vi "ValidateRule.vi"(8 "error in (no error)":errorcluster, 9 "Target":refnum<class "ILabVIEWItem.lvclass">, 11 "CDependencyItemRule in":refnum<class "CDependencyItemRule.lvclass">) -> (0 "error out":errorcluster, 1 "Pass?":bool, 2 "Is concession?":bool, 3 "CDependencyItemRule out":refnum<class "CDependencyItemRule.lvclass">)   [LabVIEW 2020, in "LabVIEWContainers.lvlib" / "CDependencyItemRule.lvclass"]
uses:
  CDependencyItemRule.lvclass
  LabVIEWObjectInterfaces/ILabVIEWItem/ILabVIEWItem.lvclass
  CommonHelpers/CommonHelpers.lvlib
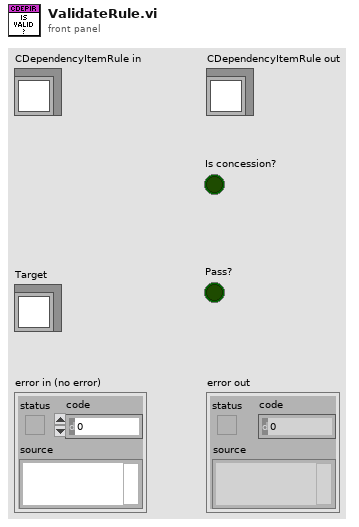
[diagram p1: front panel]
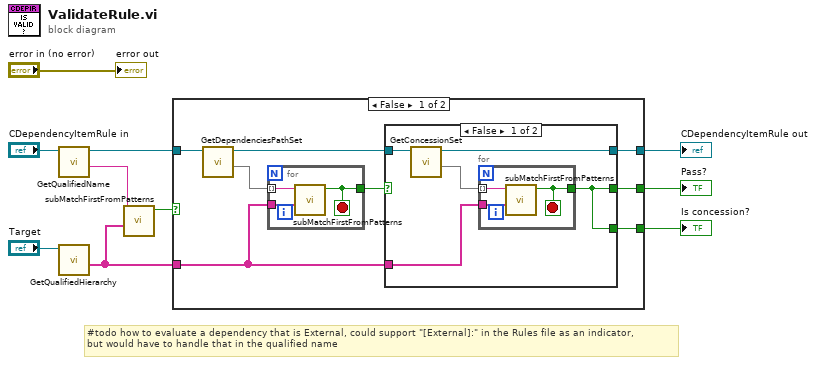
[diagram p0: block diagram]
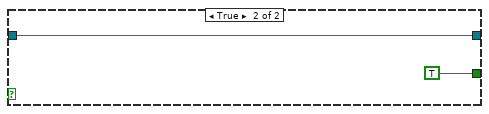
[diagram p3: hidden frame]
diagram:
  # "#todo how to evaluate a dependency that is External, could support \"[External]:\" in the Rules file as an indicator, \nbut would have to handle that in the qualified name"
  n1 = call-dynamic "GetQualifiedName.vi"("CLabVIEWItem in"="CDependencyItemRule in") -> ("Qualified name"=w3:string, "CLabVIEWItem out"=w4:refnum<class "CDependencyItemRule.lvclass">)  [unwired: 8 in, 1 out]
  n2 = call-dynamic "GetQualifiedHierarchy.vi"("ILabVIEWItem in"="Target") -> ("Qualified hierarchy"=w2:string[])  [unwired: 8 in, 2 out]
  n3 = call "subMatchFirstFromPatterns.vi"("patterns"=w2, "string in"=w3) -> ("found?"=w1:bool)  [unwired: 7 in, 2 out]
  n4 = case shown="False" w1 {
    tunnel: w4 -> [w18 w33]
    tunnel: [w16 w33] -> w9
    tunnel: [w13 TRUE ("found?")] -> w7
    tunnel: [w12 _] -> w6
    tunnel: w2 -> [w11 _]
    frame False {
      n5 = call-dynamic "GetDependenciesPathSet.vi"("CLabVIEWItem in"=w18) -> ("Dependencies"=w15:set{string}, "CLabVIEWItem out"=w17:refnum<class "CDependencyItemRule.lvclass">)  [unwired: 8 in, 1 out]
      n6 = for {
        tunnel: w15 -> [w31] mode=indexing
        tunnel: w11 -> [w30]
        tunnel: [w29] -> w14
        stop <- w29 stop-if-true
        n7 = call "subMatchFirstFromPatterns.vi"("patterns"=w30, "string in"=w31) -> ("found?"=w29:bool)  [unwired: 7 in, 2 out]
      }
      n8 = case shown="False" w14 {
        selector: w14 -> [_ w27]
        tunnel: w17 -> [w23 w28]
        tunnel: [w22 w28] -> w16
        tunnel: w11 -> [w20 _]
        tunnel: [w19 w27] -> w13
        tunnel: [w19 _] -> w12
        frame False {
          n9 = call-dynamic "GetConcessionSet.vi"("CDependencyItemRule in"=w23) -> ("Concessions"=w21:set{string}, "CDependencyItemRule out"=w22:refnum<class "CDependencyItemRule.lvclass">)  [unwired: 8 in, 1 out]
          n10 = for {
            tunnel: w21 -> [w26] mode=indexing
            tunnel: w20 -> [w25]
            tunnel: [w24] -> w19
            stop <- w24 stop-if-true
            n11 = call "subMatchFirstFromPatterns.vi"("patterns"=w25, "string in"=w26) -> ("found?"=w24:bool)  [unwired: 7 in, 2 out]
          }
        }
        frame True {
        }
      }
    }
    frame True {
    }
  }
  "CDependencyItemRule out" <- w9
  "Is concession?" <- w6
  "Pass?" <- w7
  "error out" <- "error in (no error)"
